vi "TestAiRev2.vi"() -> ()   [LabVIEW 2012]
uses:
  <vilib>/rvi/Emulation/niFpgaSctlEmulationGetInTimedLoop.vi
  glADC.vi
  <vilib>/rvi/Emulation/niFpgaSctlEmulationGlobalWrite.vi
panel:
  out "FRSTDATA 2":bool[](array[boolean])
  in  "ADC 7609":T1={"OS"=0, "Range"=1, "T_hi"=2, "D_low"=2} {"Range" items=["+-20V", "+-10V", "+-5V"]; "OS" items=["NONE", "2X", "4X", "8X", "16X", "32X", "64"]}
  out "NumReset":u32
  out "FRSTDATA":bool[](array[boolean])
  out "x-y":u32
  in  "stop":bool
  in  "AutoReset":bool
  out "DATA":i16[](array[numeric])=[9827, -1, 0, -1, -1, 1, 3, 13138, 0, 0, 0, 0, 0, 0, 0, 0]
  in  "Loop(ticks)":u32=400 caption="Count(Ticks)"
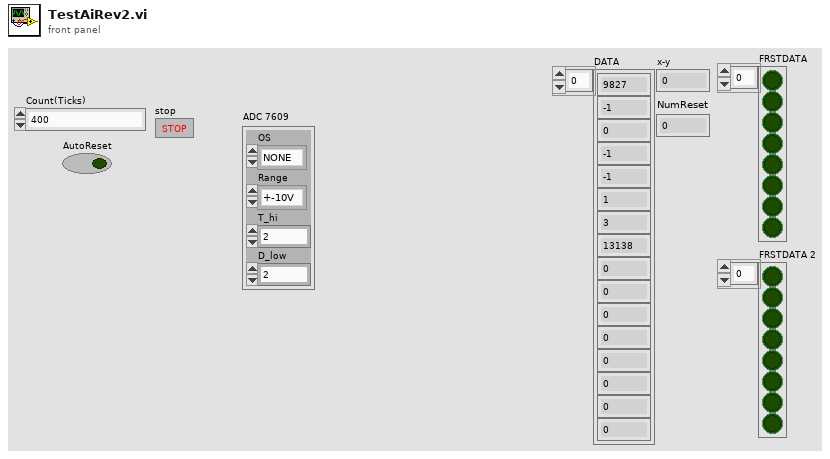
[diagram p1: front panel]
types:
  T1 = cluster{"OS":u8, "Range":u8, "T_hi":u8, "D_low":u8}
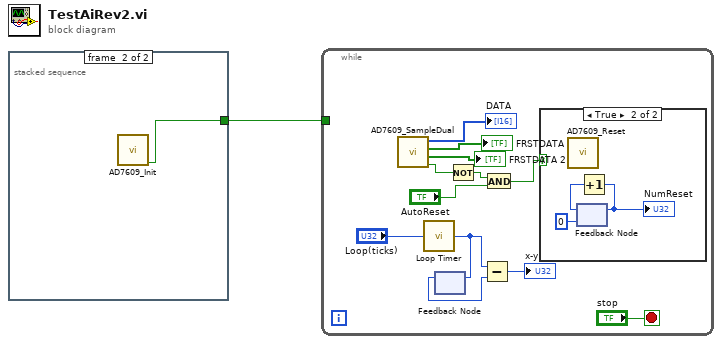
[diagram p0: block diagram]
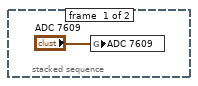
[diagram p2: hidden frame]
diagram:
  n1 = stacked-sequence {
    tunnel: [_ w3] -> w1
    frame #0 {
      n2 = global write "glADC.vi" "ADC 7609"("ADC 7609") -> ()
    }
    frame #1 {
      n3 = call "AD7609_Init.vi"() -> ("OK"=w3:bool)  [unwired: 11 in]
    }
  }
  n4 = while {
    tunnel: w1 -> [_]
    stop <- "stop" stop-if-true
    n5 = call "AD7609_SampleDual.vi"() -> ("OK"=w13:bool, "FRSTDATA 2"=→"FRSTDATA 2":bool[], "FRSTDATA"=→"FRSTDATA":bool[], "DATA"=→"DATA":i16[])  [unwired: 8 in]
    n6 = call "Loop Timer"("Count(Ticks)"="Loop(ticks)") -> ("Tick Count(Ticks)"=w8:u32)
    n7 = feedback-in #1(w8) -> ()
    n8 = feedback #1() -> (w7:u32)  [unwired: 1 in]
    n9 = Not(x=w13) -> (.not. x?=w10:bool)
    n10 = Subtract(x=w8, y=w7) -> (x-y=→"x-y":u32)
    n11 = And(x=w10, y="AutoReset") -> (x .and. y?=w11:bool)
    n12 = case shown="True" w11 {
      frame False {
      }
      frame True {
        n13 = call "AD7609_Reset.vi"() -> ()  [unwired: 12 in]
        n14 = feedback #2(u32 0) -> (w17:u32)
        n15 = Increment(x=w17) -> (x+1=w18:u32)
        "NumReset" <- w18
        n16 = feedback-in #2(w18) -> ()
      }
    }
  }
